vi "Omron Serial FINS-Example.vi"() -> ()   [LabVIEW 2016]
uses:
  Data Def/Omron Serial FINS-Connection Data.ctl
  SubVI/Omron Serial FINS-Read Data(I16 Array).vi
  SubVI/Omron Serial FINS-Read Data(I16 Element).vi
  SubVI/Omron Serial FINS-Read Data(Boolean Element).vi
  SubVI/Omron Serial FINS-Read Data(Boolean Array).vi
  SubVI/Omron Serial FINS-Write Data(I16 Array).vi
  SubVI/Omron Serial FINS-Write Data(I16 Element).vi
  SubVI/Omron Serial FINS-Write Data(Boolean Element).vi
  SubVI/Omron Serial FINS-Write Data(Boolean Array).vi
panel:
  out "Connect?":bool
  in  "Connect":bool
  in  "Connection Data":T1={"VISA Resource Name"="COM4", "Baud Rate"=115200, "Data Bits"=7, "Parity"=2, "Stop Bits"=20, "Wait For Read(ms)"=0} {"Stop Bits" items=["1.0"=10, "1.5"=15, "2.0"=20]; "Parity" items=["None", "Odd", "Even", "Mark", "Space"]}
  in  "Polling Time":i32
  out "Time":u32
  in  "Read Data":bool
  in  "Read Type":T2(tab)
  in  "Read Setting(I16 Array)":T3={"I/O Memory Address"=130, "Beginning Address"=0, "No. Of Items"=1} {"I/O Memory Address" items=["DM"=130, "CIO"=176, "WR"=177, "HR"=178, "AR"=179, "TIM"=137, "EM"=152]}
  out "Data(I16 Array)-Read":i16[](array[numeric])
  in  "Read Setting(I16 Element)":T4={"I/O Memory Address"=130, "Data Address"=0} {"I/O Memory Address" items=["DM"=130, "CIO"=176, "WR"=177, "HR"=178, "AR"=179, "TIM"=137, "EM"=152]}
  out "Data(I16 Element)-Read":i16
  in  "Read Setting(Boolean Element)":T5={"I/O Memory Address"=130, "Data Address"=0, "Bit Index"=0} {"I/O Memory Address" items=["DM"=130, "CIO"=176, "WR"=177, "HR"=178, "AR"=179, "TIM"=137, "EM"=152]}
  out "Data(Boolean Element)-Read":bool
  in  "Read Setting(Boolean Array)":T4={"I/O Memory Address"=130, "Data Address"=0} {"I/O Memory Address" items=["DM"=130, "CIO"=176, "WR"=177, "HR"=178, "AR"=179, "TIM"=137, "EM"=152]}
  out "Data(Boolean Array)-Read":bool[](array[boolean])
  in  "Write Type":T2(tab)
  in  "Write Setting(I16 Array)":T3={"I/O Memory Address"=130, "Beginning Address"=0, "No. Of Items"=1} {"I/O Memory Address" items=["DM"=130, "CIO"=176, "WR"=177, "HR"=178, "AR"=179, "TIM"=137, "EM"=152]}
  in  "Data(I16 Array)-Write":i16[](array[numeric])=[0]
  in  "Write Setting(I16 Element)":T4={"I/O Memory Address"=130, "Data Address"=0} {"I/O Memory Address" items=["DM"=130, "CIO"=176, "WR"=177, "HR"=178, "AR"=179, "TIM"=137, "EM"=152]}
  in  "Data(I16 Element)-Write":i16
  in  "Write Setting(Boolean Element)":T5={"I/O Memory Address"=130, "Data Address"=0, "Bit Index"=0} {"I/O Memory Address" items=["DM"=130, "CIO"=176, "WR"=177, "HR"=178, "AR"=179, "TIM"=137, "EM"=152]}
  in  "Data(Boolean Element)-Write":bool
  in  "Write Setting(Boolean Array)":T4={"I/O Memory Address"=130, "Data Address"=0} {"I/O Memory Address" items=["DM"=130, "CIO"=176, "WR"=177, "HR"=178, "AR"=179, "TIM"=137, "EM"=152]}
  in  "Data(Boolean Array)-Write":bool[](array[boolean])=[FALSE, FALSE, FALSE, FALSE, FALSE, FALSE, FALSE, FALSE, FALSE, FALSE, FALSE, FALSE, FALSE, FALSE, FALSE, FALSE]
  in  "Write Data":bool
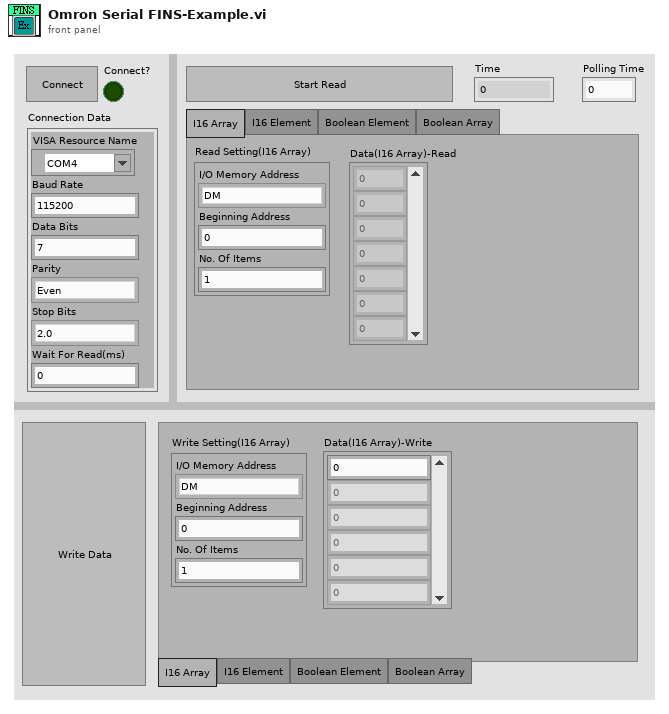
[diagram p1: front panel]
types:
  T1 = typedef "Omron Serial FINS-Connection Data.ctl" = cluster{"VISA Resource Name":refnum<visa-resource-name>, "Baud Rate":u32, "Data Bits":u16, "Parity":u16, "Stop Bits":u16, "Wait For Read(ms)":u32}
  T2 = enum32{"I16 Array", "I16 Element", "Boolean Element", "Boolean Array"}
  T3 = cluster{"I/O Memory Address":i32, "Beginning Address":u32, "No. Of Items":u32}
  T4 = cluster{"I/O Memory Address":i32, "Data Address":u32}
  T5 = cluster{"I/O Memory Address":i32, "Data Address":u32, "Bit Index":i32}
  T6 = typedef "Omron Serial FINS-Buffer Data.ctl" = cluster{"VISA Resource Name":refnum<visa-resource-name>, "Wait For Read(ms)":u32, "Command Code":T7, "Command String":string, "Read Bytes":u32, "Response String":string}
  T7 = typedef "Omron Serial FINS-Command Code.ctl" = enum16{"Memory area read", "Memory area write"}
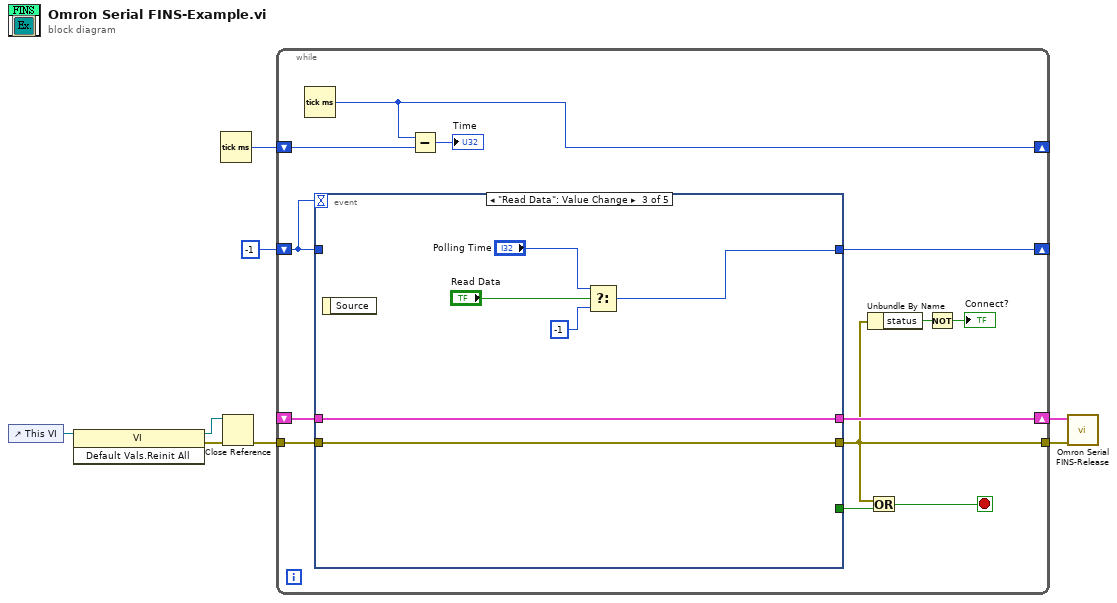
[diagram p0: block diagram]
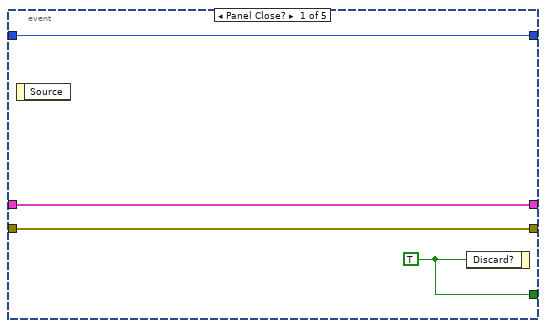
[diagram p2: hidden frame]
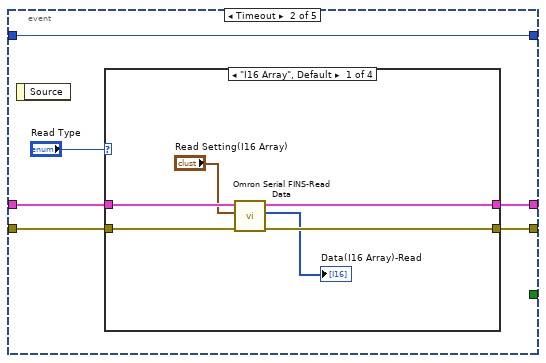
[diagram p3: hidden frame]
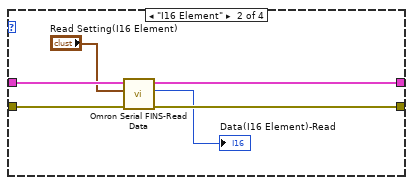
[diagram p4: hidden frame]
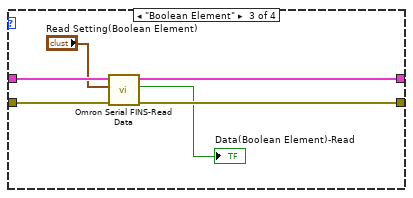
[diagram p5: hidden frame]
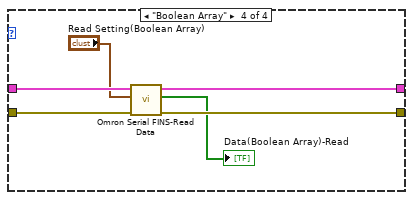
[diagram p6: hidden frame]
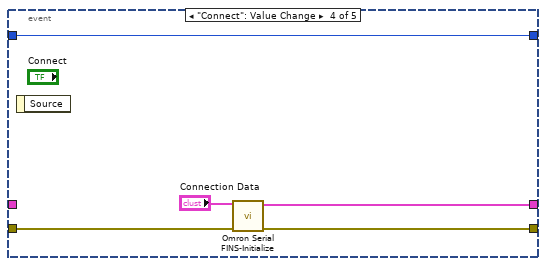
[diagram p7: hidden frame]
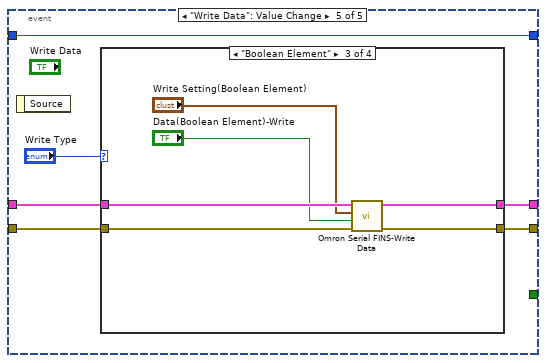
[diagram p8: hidden frame]
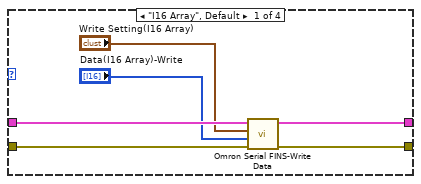
[diagram p9: hidden frame]
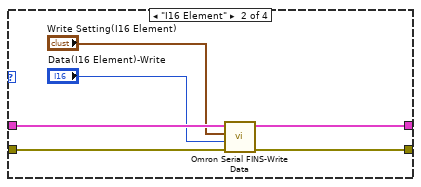
[diagram p10: hidden frame]
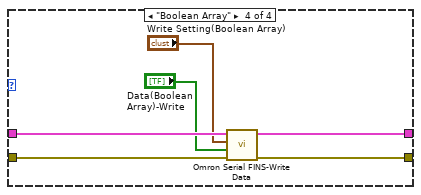
[diagram p11: hidden frame]
diagram:
  n1 = control-ref of="This VI"() -> (w5:refnum<vi>)
  n2 = invoke class="VI" method="Default Vals.Reinit All"(reference=w5) -> (reference out=w3:refnum<vi>, error out=w4:errorcluster)  [unwired: 2 in, 1 out]
  n3 = Tick Count (ms)() -> (millisecond timer value=w1:u32)
  n4 = Close Reference(reference=w3, error in (no error)=w4) -> (error out=w2:errorcluster)
  n5 = while {
    tunnel: w2 -> [w20]
    shift-right: [w17] -> w8
    shift-left: _ -> [w21]
    shift-right: [w18] -> _
    shift-left: -1 -> [w19]
    tunnel: [w14] -> w6
    shift-right: [w11] -> _
    shift-left: w1 -> [w10]
    stop <- w15 stop-if-true
    n6 = Tick Count (ms)() -> (millisecond timer value=w11:u32)
    n7 = event shown="[2] \"Read Data\": Value Change" {
      selector: _ -> [_ _ _ _ _]
      dyn-events: _ -> [_ _ _ _ _]
      timeout: w19 -> [_ _ _ _ _]
      tunnel: w21 -> [w24 w29 w60 _ w70]
      tunnel: w20 -> [w23 w28 w57 w64 w69]
      tunnel: w19 -> [w25 w31 _ w66 w72]
      tunnel: [w25 w31 w59 w66 w72] -> w18
      tunnel: [w24 w26 w60 w63 w68] -> w17
      tunnel: [w23 w27 w57 w62 w67] -> w14
      tunnel: [w22 _ _ _ _] -> w16
      event Panel Close? {
        w22 = TRUE ("Discard?")
        n8 = event-data() -> ()  [unwired: 1 in, 1 out]
        n9 = event-data("Discard?"=w22) -> ()  [unwired: 1 in, 1 out]
      }
      event Timeout {
        n10 = event-data() -> ()  [unwired: 1 in, 1 out]
        n11 = case shown="\"I16 Array\", Default" "Read Type" {
          tunnel: w29 -> [w37 w43 w49 w55]
          tunnel: w28 -> [w36 w42 w48 w54]
          tunnel: [w35 w41 w47 w53] -> w27
          tunnel: [w34 w40 w46 w52] -> w26
          frame "I16 Array", Default {
            n12 = call-poly "Omron Serial FINS-Read Data.vi"("error in"=w36, "Read Setting(I16 Array)"="Read Setting(I16 Array)", "Buffer Data In"=w37) -> ("error out"=w35:errorcluster, "Data"=→"Data(I16 Array)-Read":i16[], "Buffer Data Out"=w34:T6)  [unwired: 6 in]
          }
          frame "I16 Element" {
            n13 = call-poly "Omron Serial FINS-Read Data.vi"("error in"=w42, "Read Setting(I16 Element)"="Read Setting(I16 Element)", "Buffer Data In"=w43) -> ("error out"=w41:errorcluster, "Data"=→"Data(I16 Element)-Read":i16, "Buffer Data Out"=w40:T6)  [unwired: 6 in]
          }
          frame "Boolean Element" {
            n14 = call-poly "Omron Serial FINS-Read Data.vi"("error in"=w48, "Read Setting(Boolean Element)"="Read Setting(Boolean Element)", "Buffer Data In"=w49) -> ("error out"=w47:errorcluster, "Data"=→"Data(Boolean Element)-Read":bool, "Buffer Data Out"=w46:T6)  [unwired: 6 in]
          }
          frame "Boolean Array" {
            n15 = call-poly "Omron Serial FINS-Read Data.vi"("error in"=w54, "Read Setting(Boolean Array)"="Read Setting(Boolean Array)", "Buffer Data In"=w55) -> ("error out"=w53:errorcluster, "Data"=→"Data(Boolean Array)-Read":bool[], "Buffer Data Out"=w52:T6)  [unwired: 6 in]
          }
        }
      }
      event "Read Data": Value Change {
        n16 = event-data() -> ()  [unwired: 1 in, 1 out]
        n17 = Select(t="Polling Time", s="Read Data", f=-1) -> (s? t:f=w59:i32)
      }
      event "Connect": Value Change {
        n18 = event-data() -> ()  [unwired: 1 in, 1 out]
        n19 = call "Omron Serial FINS-Initialize.vi"("error in"=w64, "Connection Data In"="Connection Data") -> ("error out"=w62:errorcluster, "Buffer Data"=w63:T6)  [unwired: 8 in]
      }
      event "Write Data": Value Change {
        n20 = event-data() -> ()  [unwired: 1 in, 1 out]
        n21 = case shown="\"Boolean Element\"" "Write Type" {
          tunnel: w70 -> [w78 w83 w90 w96]
          tunnel: w69 -> [w77 w84 w86 w95]
          tunnel: [w75 w82 w89 w94] -> w68
          tunnel: [w76 w81 w85 w93] -> w67
          frame "I16 Array", Default {
            n22 = call-poly "Omron Serial FINS-Write Data.vi"("error in"=w77, "Data"="Data(I16 Array)-Write", "Write Setting(I16 Array)"="Write Setting(I16 Array)", "Buffer Data In"=w78) -> ("error out"=w76:errorcluster, "Buffer Data Out"=w75:T6)  [unwired: 6 in]
          }
          frame "I16 Element" {
            n23 = call-poly "Omron Serial FINS-Write Data.vi"("error in"=w84, "Data"="Data(I16 Element)-Write", "Write Setting(I16 Element)"="Write Setting(I16 Element)", "Buffer Data In"=w83) -> ("error out"=w81:errorcluster, "Buffer Data Out"=w82:T6)  [unwired: 6 in]
          }
          frame "Boolean Element" {
            n24 = call-poly "Omron Serial FINS-Write Data.vi"("error in"=w86, "Data"="Data(Boolean Element)-Write", "Write Setting(Boolean Element)"="Write Setting(Boolean Element)", "Buffer Data In"=w90) -> ("error out"=w85:errorcluster, "Buffer Data Out"=w89:T6)  [unwired: 6 in]
          }
          frame "Boolean Array" {
            n25 = call-poly "Omron Serial FINS-Write Data.vi"("error in"=w95, "Data"="Data(Boolean Array)-Write", "Write Setting(Boolean Array)"="Write Setting(Boolean Array)", "Buffer Data In"=w96) -> ("error out"=w93:errorcluster, "Buffer Data Out"=w94:T6)  [unwired: 6 in]
          }
        }
      }
    }
    n26 = Subtract(x=w11, y=w10) -> (x-y=→"Time":u32)
    n27 = Unbundle By Name(w14) -> ("status"=w13:bool)
    n28 = Or(x=w14, y=w16) -> (x .or. y?=w15:bool)
    n29 = Not(x=w13) -> (.not. x?=→"Connect?":bool)
  }
  n30 = call "Omron Serial FINS-Release.vi"("error in"=w6, "Buffer Data"=w8) -> ()  [unwired: 9 in, 1 out]
